vi "Stop.vi"(8 "error in":errorcluster, 11 "Copy of PCAN in":refnum<class "PCAN.lvclass">) -> (0 "error out":errorcluster, 3 "Copy of PCAN out":refnum<class "PCAN.lvclass">)   [LabVIEW 2024, in "PCAN.lvlib" / "PCAN.lvclass"]
uses:
  PCAN.lvclass
  PCAN.lvclass/PCAN.ctl
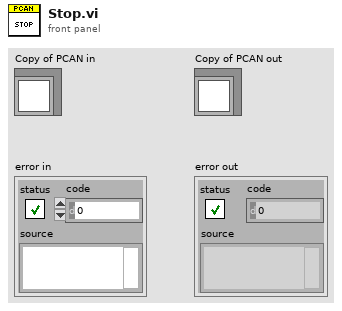
[diagram p1: front panel]
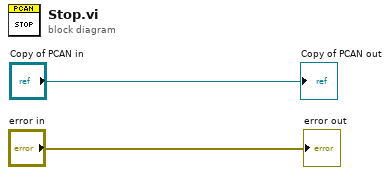
[diagram p0: block diagram]
diagram:
  "error out" <- "error in"
  "Copy of PCAN out" <- "Copy of PCAN in"
